vi "TTLDisconnect.vi"(2 "error in":errorcluster, 3 "socket in":refnum<class "zmq_socket.lvclass">, 4 "context in":refnum<class "zmq_context.lvclass">) -> (0 "error out":errorcluster)   [LabVIEW 2017]
doc: "Safely disconnects and closes a ZeroMQ socket."
uses:
  <vilib>/addons/zeromq/zmq_socket.lvclass
  <vilib>/addons/zeromq/zmq_context.lvclass
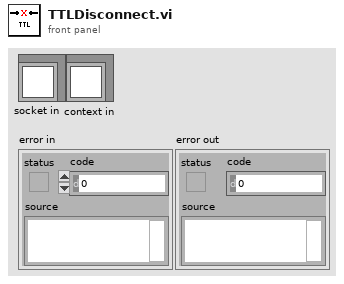
[diagram p1: front panel]
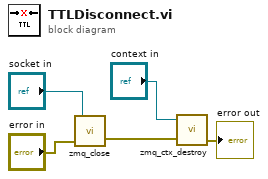
[diagram p0: block diagram]
diagram:
  n1 = call <vilib>:"zmq_close.vi"("error in"="error in", "socket"="socket in") -> ("error out"=w5:errorcluster)  [unwired: 3 in]
  n2 = call <vilib>:"zmq_ctx_destroy.vi"("error in"=w5, "context in"="context in") -> ("error out"=→"error out":errorcluster)  [unwired: 3 in]
